vi "Create Dummy Country Data.vi"(8 "error in (no error)":errorcluster) -> (0 "error out":errorcluster, 3 "Country":refnum<class "Country.lvclass">)   [LabVIEW 2017, in "Generic Object Serializer Tests.lvlib"]
uses:
  Generic Object Serializer Tests.lvlib
  Country/Country.lvclass
  City/City.lvclass
  Weather Forecast/Weather Forecast.lvclass
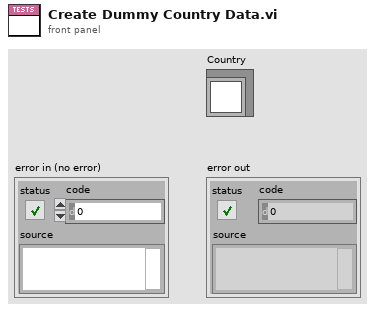
[diagram p1: front panel]
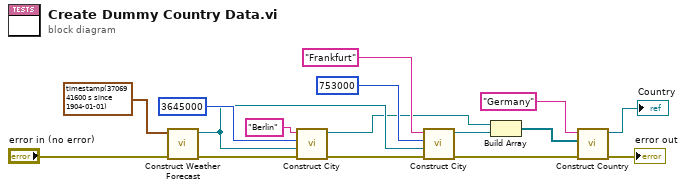
[diagram p0: block diagram]
diagram:
  n1 = call "Construct Weather Forecast.vi"("error in (no error)"="error in (no error)", "Date"=timestamp(3706941600 s since 1904-01-01)) -> ("error out"=w10:errorcluster, "Weather Forecast"=w9:refnum<class "Weather Forecast.lvclass">)  [unwired: 8 in]
  n2 = call "Construct City.vi"("error in (no error)"=w10, "Weather Forecast"=w9, "Population"=u32 3645000, "Name"="Berlin") -> ("error out"=w13:errorcluster, "City"=w6:refnum<class "City.lvclass">)  [unwired: 6 in]
  n3 = call "Construct City.vi"("error in (no error)"=w13, "Weather Forecast"=w9, "Population"=u32 753000, "Name"="Frankfurt") -> ("error out"=w4:errorcluster, "City"=w7:refnum<class "City.lvclass">)  [unwired: 6 in]
  n4 = Build Array(w6, w7) -> (w8:refnum<class "City.lvclass">[])
  n5 = call "Construct Country.vi"("error in (no error)"=w4, "Cities"=w8, "Name"="Germany") -> ("error out"=→"error out":errorcluster, "Country"=→"Country":refnum<class "Country.lvclass">)  [unwired: 7 in]
